vi "HTTP URL Generator.vi"() -> ()   [LabVIEW 2014]
uses:
  Shared/Controls/LabVIEW Build - STYP.ctl
  <vilib>/wsapi/NI_WebServices.lvlib
panel:
  in  "IP Address (Not Localhost)":string="10.211.55.18"
  out "URL":string
  in  "Tab Control":enum32{"LabVIEW EXE Build", "Page 2"}(tab)
  in  "Workspace Path":path=path "C:/Program Files (x86)/Jenkins/jobs/Test LabVIEW CI Service/workspace"
  in  "Build Spec":string="LabVIEW CI Service"
  in  "Project Path":path=path "C:/Projects/LabVIEW Continuous Integration/LabVIEW Continuous Integration.lvproj"
  in  "Auto Increment Version?":bool
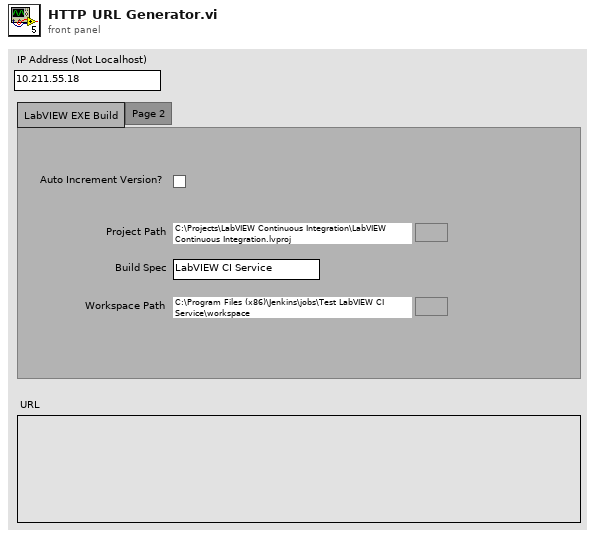
[diagram p1: front panel]
types:
  T1 = typedef "LabVIEW Build - STYP.ctl" = cluster{"Executor_Number":string, "Workspace_Path":string, "Build_Spec":string, "Project_Path":string, "Auto_Version_Increment":bool}
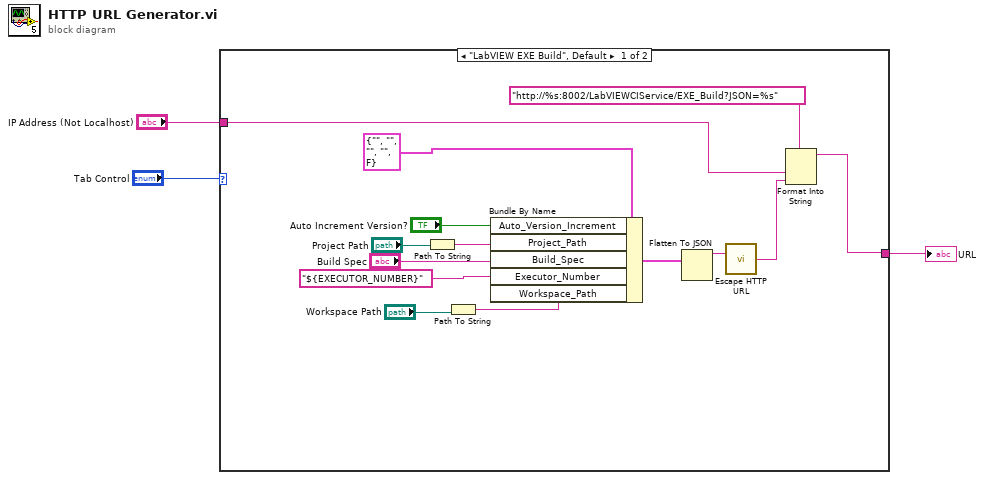
[diagram p0: block diagram]
diagram:
  n1 = case shown="\"LabVIEW EXE Build\", Default" "Tab Control" {
    tunnel: [w9 _] -> w2
    tunnel: "IP Address (Not Localhost)" -> [w10 _]
    frame "LabVIEW EXE Build", Default {
      n2 = Path To String(path="Project Path") -> (string=w15:string)
      n3 = Path To String(path="Workspace Path") -> (string=w7:string)
      n4 = Bundle By Name(cluster=T1 {"Executor_Number"="", "Workspace_Path"="", "Build_Spec"="", "Project_Path"="", "Auto_Version_Increment"=FALSE} ("LabVIEW Build"), "Auto_Version_Increment"="Auto Increment Version?", "Project_Path"=w15, "Build_Spec"="Build Spec", "Executor_Number"="${EXECUTOR_NUMBER}", "Workspace_Path"=w7) -> (w13:T1)
      n5 = Flatten To JSON(anything=w13) -> (JSON string=w5:string)  [unwired: 2 in, 1 out]
      n6 = call <vilib>:"Escape HTTP URL.vi"("unescaped string in"=w5) -> ("escaped string out"=w4:string)
      n7 = Format Into String(format string="http://%s:8002/LabVIEWCIService/EXE_Build?JSON=%s", w10, w4) -> (resulting string=w9:string)  [unwired: 2 in, 1 out]
    }
    frame "Page 2" {
    }
  }
  "URL" <- w2
